vi "send_vehicle_control_command.vi"(6 "manual_gear":T1={"use_manual_gear"=TRUE, "gear"=2} {"gear" min=-1 max=5 step=1}, 7 "vehicle":string="crossover", 8 "error in":errorcluster, 9 "set_manual_control_mode_pedal":bool, 10 "Vehicle control":T2, 11 "auto_pilot_control":T3={"debug_drawing"=FALSE, "desired_speed"=0, "destroy_on_collision"=TRUE, "ignore_lane_change_boxes"=FALSE, "ignore_other_vehicles"=FALSE, "ignore_traffic_signals"=FALSE, "lane_change"=0, "lane_change_safe"=TRUE, "lane_offset"=0, "obey_road_speed_limits"=TRUE, "search_backward_distance"=10000, "search_forward_distance"=15000, "set_auto_control_mode"=FALSE, "set_debug_drawing"=FALSE, "set_desired_speed"=FALSE, "set_destroy_on_collision"=FALSE, "set_ignore_lane_change_boxes"=FALSE, "set_ignore_other_vehicles"=FALSE, "set_ignore_traffic_signals"=FALSE, "set_lane_change"=FALSE, "set_lane_change_safe"=FALSE, "set_lane_offset"=FALSE, "set_obey_speed_limits"=FALSE, "set_search_backward_distance"=FALSE, "set_search_forward_distance"=FALSE, "set_show_vehicle_charts"=FALSE, "set_turn_preference"=FALSE, "show_vehicle_charts"=FALSE, "turn_preference"=3, "set_limit_speed_in_curves"=FALSE, "limit_speed_in_curves"=TRUE}) -> (0 "error out":errorcluster, 3 "success":bool)   [LabVIEW 2019, in "Lib_Simx.lvlib"]
uses:
  Lib_Simx.lvlib
  controls/AutoPilot.ctl
  controls/Manual Gear.ctl
  controls/VehicleControl.ctl
  tools/simx_common.vi
panel:
  out "TCP Network Connection out":refnum<k5>
  out "Vehicle command response":string
  # "Autopilot Control"
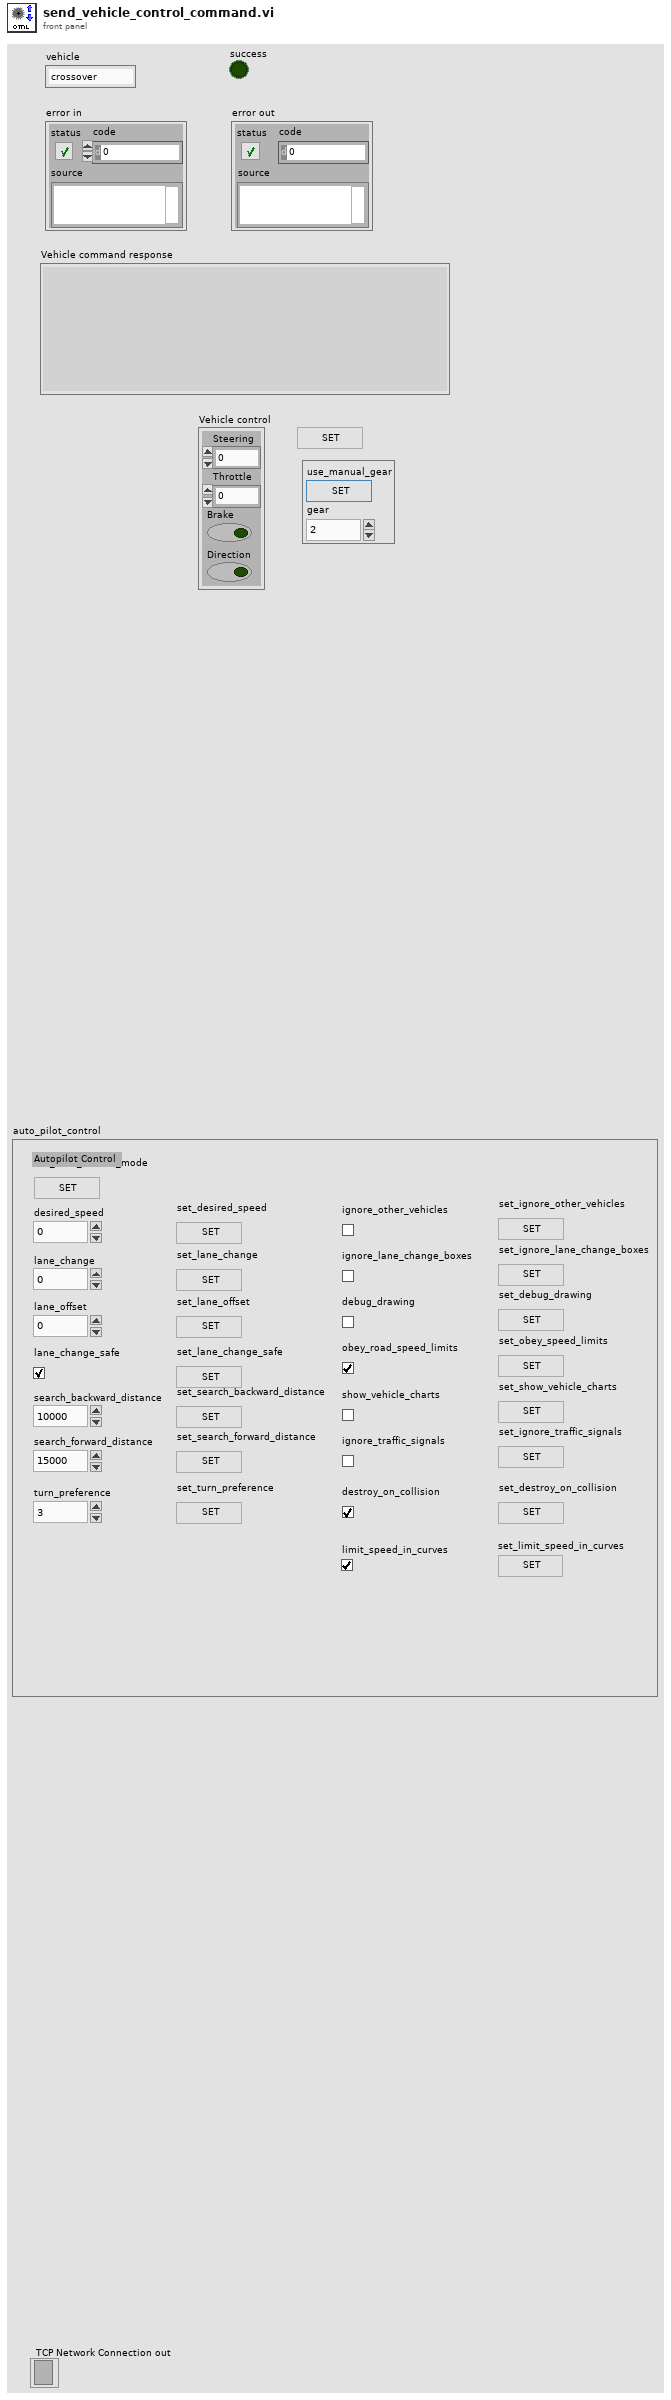
[diagram p1: front panel]
types:
  T1 = typedef "Lib_Simx.lvlib/Manual Gear.ctl" = cluster{"use_manual_gear":bool, "gear":i32}
  T2 = cluster{"Steering":sgl, "Throttle":sgl, "Brake":bool, "Direction":bool}
  T3 = typedef "Lib_Simx.lvlib/AutoPilot.ctl" = cluster{"debug_drawing":bool, "desired_speed":i32, "destroy_on_collision":bool, "ignore_lane_change_boxes":bool, "ignore_other_vehicles":bool, "ignore_traffic_signals":bool, "lane_change":i32, "lane_change_safe":bool, "lane_offset":i32, "obey_road_speed_limits":bool, "search_backward_distance":i32, "search_forward_distance":i32, "set_auto_control_mode":bool, "set_debug_drawing":bool, "set_desired_speed":bool, "set_destroy_on_collision":bool, "set_ignore_lane_change_boxes":bool, "set_ignore_other_vehicles":bool, "set_ignore_traffic_signals":bool, "set_lane_change":bool, "set_lane_change_safe":bool, "set_lane_offset":bool, "set_obey_speed_limits":bool, "set_search_backward_distance":bool, "set_search_forward_distance":bool, "set_show_vehicle_charts":bool, "set_turn_preference":bool, "show_vehicle_charts":bool, "turn_preference":i32, "set_limit_speed_in_curves":bool, "limit_speed_in_curves":bool}
  T4 = typedef "Lib_Simx.lvlib/simx_connection.ctl" = cluster{"Config":T5, "Connections":T8, "Map":cluster{"lanes":cluster{"x":dbl[], "y":dbl[], "z":dbl[]}, "StartPosition":cluster{"start_points":T9, "StartRotation":dbl[], "StartLocation":dbl[]}, "Draw Map Size":T10, "DrawArea":cluster{"min_Y":dbl, "min_X":dbl, "Scale X":dbl, "Scale Y":dbl}, "Map":picture, "Map Geojson":string}}
  T5 = typedef "Lib_Simx.lvlib/config.ctl" = cluster{"Trajectory":T6, "Weather":T7}
  T6 = typedef "Lib_Simx.lvlib/trajectory.ctl" = cluster{"Number of frames":i32, "Frame number":i32, "Trajectory":string}
  T7 = typedef "Lib_Simx.lvlib/weather.ctl" = cluster{"id":string}
  T8 = typedef "Lib_Simx.lvlib/connections.ctl" = cluster{"Simulator Connection":refnum<k5>, "server_ip":string, "Port":i32, "Sensor connections":refnum<k5>[]}
  T9 = typedef "Lib_Simx.lvlib/start_points.ctl" = cluster{"locations":dbl[][], "rotations":dbl[][], "type":string[]}
  T10 = typedef "LVBoundsTypeDef.ctl" = cluster{"Width":u32, "Height":u32}
  T11 = typedef "Lib_Simx.lvlib/VehicleControl.ctl" = cluster{"auto_pilot_control":T3, "manual_control":cluster{"brake_amount":sgl, "brake_torque":sgl[][], "drive_mode":i16, "drive_torque":sgl[][], "forward_amount":sgl, "manual_gear":cluster{"gear":i32, "use_manual_gear":bool}, "right_amount":sgl, "set_manual_control_mode_pedal":bool, "set_manual_control_mode_torque":bool, "steer_angle":sgl[][]}, "vehicle":string}
  T12 = typedef "Lib_Simx.lvlib/Manual Control.ctl" = cluster{"set_manual_control_mode_pedal":bool, "Torque Control":T13, "manual_gear":T1, "right_amount":sgl, "forward_amount":sgl, "brake_amount":sgl, "drive_mode":i16}
  T13 = typedef "Lib_Simx.lvlib/TorqueControlVehicle.ctl" = cluster{"set_manual_control_mode_torque":bool, "steer_angle":sgl[][], "drive_torque":sgl[][], "brake_torque":sgl[][]}
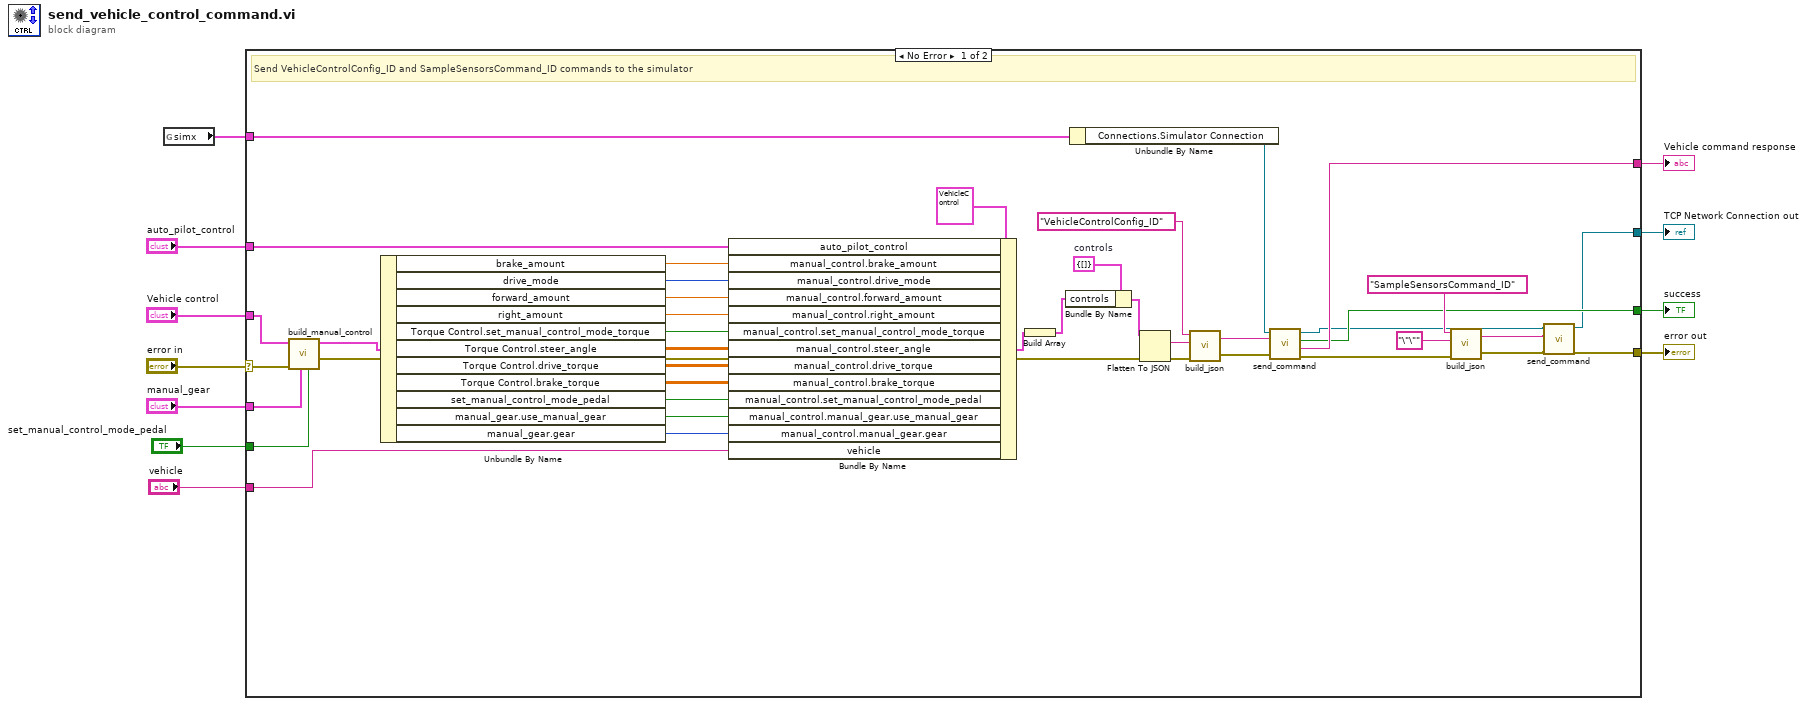
[diagram p0: block diagram]
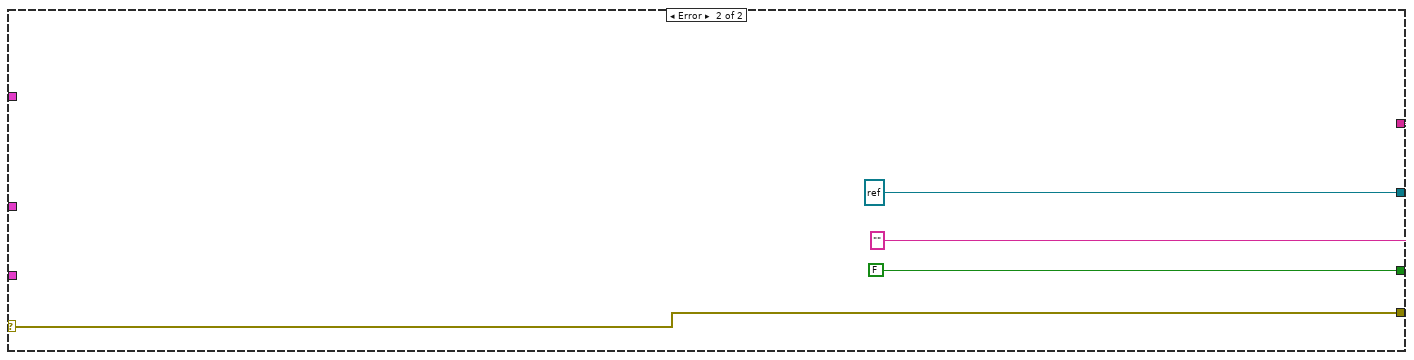
[diagram p2: hidden frame]
diagram:
  n1 = global read "simx_common.vi" "simx"() -> (w6:T4)
  n2 = case shown="No Error" "error in" {
    selector: "error in" -> [w15 w56]
    tunnel: [w35 w56] -> w11
    tunnel: [w47 "" ("response")] -> w10
    tunnel: [w34 refnum<k5> refnum ("TCP Network Connection Out")] -> w9
    tunnel: [w41 FALSE ("success")] -> w8
    tunnel: w6 -> [w52 _]
    tunnel: "auto_pilot_control" -> [w37 _]
    tunnel: "vehicle" -> [w18 _]
    tunnel: "set_manual_control_mode_pedal" -> [w13 _]
    tunnel: "Vehicle control" -> [w12 _]
    tunnel: "manual_gear" -> [w14 _]
    frame No Error {
      w39 = cluster{"controls":T11[]} {"controls"=[]}  # controls
      # "Send VehicleControlConfig_ID and SampleSensorsCommand_ID commands to the simulator"
      n3 = call "build_manual_control.vi"("set_manual_control_mode_pedal"=w13, "manual_gear"=w14, "error in"=w15, "Vehicle Control"=w12) -> ("error out"=w16:errorcluster, "manual_control"=w17:T12)  [unwired: 6 in]
      n4 = Unbundle By Name(w17) -> ("brake_amount"=w31:sgl, "drive_mode"=w30:i16, "forward_amount"=w29:sgl, "right_amount"=w28:sgl, "Torque Control.set_manual_control_mode_torque"=w24:bool, "Torque Control.steer_angle"=w25:sgl[][], "Torque Control.drive_torque"=w26:sgl[][], "Torque Control.brake_torque"=w27:sgl[][], "set_manual_control_mode_pedal"=w23:bool, "manual_gear.use_manual_gear"=w19:bool, "manual_gear.gear"=w20:i32)
      n5 = Bundle By Name(cluster=T11 {"auto_pilot_control"={"debug_drawing"=FALSE, "desired_speed"=0, "destroy_on_collision"=TRUE, "ignore_lane_change_boxes"=FALSE, "ignore_other_vehicles"=FALSE, "ignore_traffic_signals"=FALSE, "lane_change"=0, "lane_change_safe"=TRUE, "lane_offset"=0, "obey_road_speed_limits"=TRUE, "search_backward_distance"=10000, "search_forward_distance"=15000, "set_auto_control_mode"=FALSE, "set_debug_drawing"=FALSE, "set_desired_speed"=FALSE, "set_destroy_on_collision"=FALSE, "set_ignore_lane_change_boxes"=FALSE, "set_ignore_other_vehicles"=FALSE, "set_ignore_traffic_signals"=FALSE, "set_lane_change"=FALSE, "set_lane_change_safe"=FALSE, "set_lane_offset"=FALSE, "set_obey_speed_limits"=FALSE, "set_search_backward_distance"=FALSE, "set_search_forward_distance"=FALSE, "set_show_vehicle_charts"=FALSE, "set_turn_preference"=FALSE, "show_vehicle_charts"=FALSE, "turn_preference"=3, "set_limit_speed_in_curves"=FALSE, "limit_speed_in_curves"=TRUE}, "manual_control"={"brake_amount"=0.0, "brake_torque"=[[0.0, 0.0], [1.0, 0.0], [2.0, 0.0], [3.0, 0.0]], "drive_mode"=1, "drive_torque"=[[0.0, 0.0], [1.0, 0.0], [2.0, 0.0], [3.0, 0.0]], "forward_amount"=0.0, "manual_gear"={"gear"=2, "use_manual_gear"=TRUE}, "right_amount"=0.0, "set_manual_control_mode_pedal"=TRUE, "set_manual_control_mode_torque"=FALSE, "steer_angle"=[[0.0, 0.0], [1.0, 0.0], [2.0, 0.0], [3.0, 0.0]]}, "vehicle"=""} ("VehicleControl"), "auto_pilot_control"=w37, "manual_control.brake_amount"=w31, "manual_control.drive_mode"=w30, "manual_control.forward_amount"=w29, "manual_control.right_amount"=w28, "manual_control.set_manual_control_mode_torque"=w24, "manual_control.steer_angle"=w25, "manual_control.drive_torque"=w26, "manual_control.brake_torque"=w27, "manual_control.set_manual_control_mode_pedal"=w23, "manual_control.manual_gear.use_manual_gear"=w19, "manual_control.manual_gear.gear"=w20, "vehicle"=w18) -> (w22:T11)
      n6 = Build Array(w22) -> (w21:T11[])
      n7 = Bundle By Name(cluster=w39, "controls"=w21) -> (w38:cluster{"controls":T11[]})
      n8 = Unbundle By Name(w52) -> ("Connections.Simulator Connection"=w50:refnum<k5>)
      n9 = Flatten To JSON(anything=w38, error in (no error)=w16) -> (JSON string=w43:string, 11:w44:errorcluster)  [unwired: 1 in]
      n10 = call "build_json.vi"("error in"=w44, "Message"=w43, "Command_ID"="VehicleControlConfig_ID") -> ("error out"=w51:errorcluster, "JSON Out"=w49:string)  [unwired: 1 in]
      n11 = call "send_command.vi"("error in"=w51, "JSON Command"=w49, "TCP Network Connection in"=w50) -> ("error out"=w48:errorcluster, "Response"=w47:string, "Success"=w41:bool, "TCP Network Connection Out"=w33:refnum<k5>)  [unwired: 1 in]
      n12 = call "build_json.vi"("error in"=w48, "Message"="\"\"" ("message"), "Command_ID"="SampleSensorsCommand_ID" ("type")) -> ("error out"=w36:errorcluster, "JSON Out"=w32:string)  [unwired: 1 in]
      n13 = call "send_command.vi"("error in"=w36, "JSON Command"=w32, "TCP Network Connection in"=w33) -> ("error out"=w35:errorcluster, "TCP Network Connection Out"=w34:refnum<k5>)  [unwired: 1 in, 2 out]
    }
    frame Error {
    }
  }
  "Vehicle command response" <- w10
  "TCP Network Connection out" <- w9
  "error out" <- w11
  "success" <- w8
